vi "Log Data.vi"(6 "Edge indexies":i32[](array[numeric]), 8 "error in (no error)":errorcluster, 9 "Volatge":cdb[](array[numeric]), 10 "Frequency":dbl[](array[numeric]), 11 "Spectrum Recorder in":refnum<class "Spectrum Recorder too.lvclass">) -> (0 "error out":errorcluster, 3 "Spectrum Recorder out":refnum<class "Spectrum Recorder too.lvclass">)   [LabVIEW 2016, in "Spectrum Recorder too.lvclass"]
uses:
  Spectrum Recorder too.lvclass
  Spectrum Recorder too.lvclass/Spectrum Recorder too.ctl
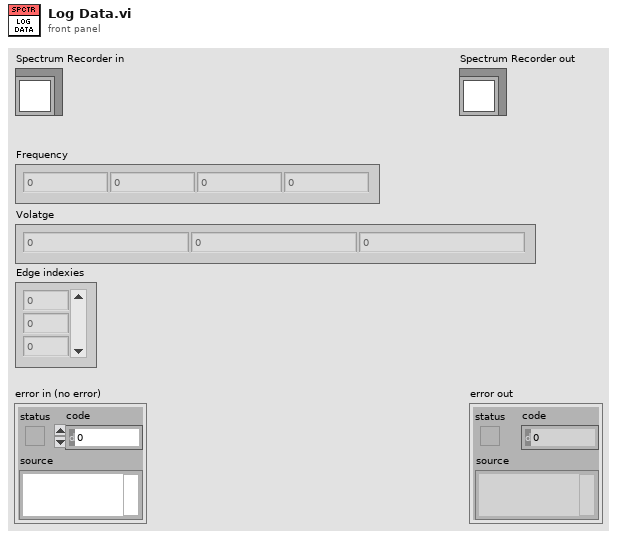
[diagram p1: front panel]
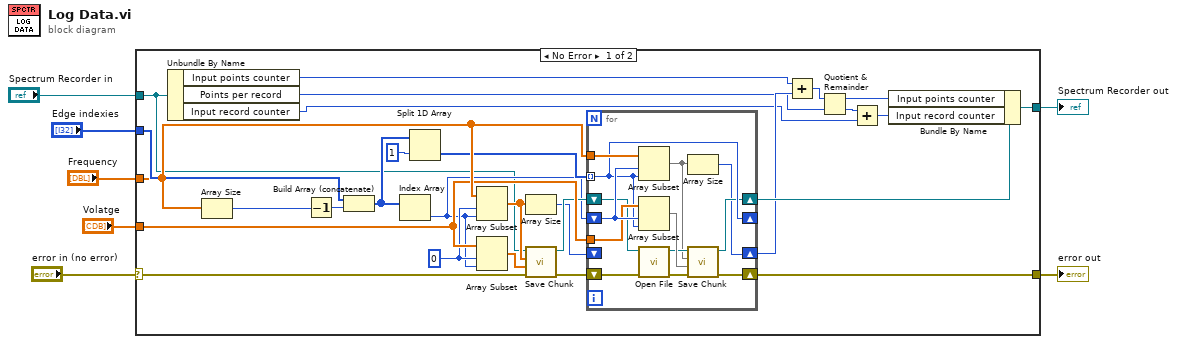
[diagram p0: block diagram]
diagram:
  n1 = case shown="No Error" "error in (no error)" {
    selector: "error in (no error)" -> [w25 w50]
    tunnel: [w31 w50] -> w6
    tunnel: [w19 w49] -> w4
    tunnel: "Spectrum Recorder in" -> [w16 w49]
    tunnel: "Edge indexies" -> [w33 _]
    tunnel: "Volatge" -> [w28 _]
    tunnel: "Frequency" -> [w29 _]
    frame No Error {
      w21 = 0
      n2 = Unbundle By Name(w16) -> ("Input points counter"=w15:i32, "Points per record"=w12:i32, "Input record counter"=w10:i32)
      n3 = Array Size(array=w29) -> (size(s)=w35:i32)
      n4 = Decrement(x=w35) -> (x-1=w34:i32)
      n5 = Build Array (concatenate)(w33, w34) -> (w27:i32[])
      n6 = Index Array(array=w27) -> (element=w20:i32)  [unwired: 1 in]
      n7 = Split 1D Array(array=w27, index=1) -> (second subarray=w23:i32[])  [unwired: 1 out]
      n8 = Array Subset(array=w29, index=w21, length=w20) -> (w17:dbl[])
      n9 = Array Subset(array=w28, index=w21, length=w20) -> (w30:cdb[])
      n10 = Array Size(array=w17) -> (size(s)=w18:i32)
      n11 = call-dynamic "Save Chunk.vi"("error in (no error)"=w25, "Voltage"=w30, "Frequency"=w17, "Spectrum Recorder in"=w16) -> ("error out"=w24:errorcluster, "Spectrum Recorder out"=w26:refnum<class "Spectrum Recorder too.lvclass">)  [unwired: 6 in]
      n12 = for {
        shift-right: [w38] -> w31
        shift-left: w24 -> [w44]
        tunnel: w29 -> [w48]
        tunnel: w28 -> [w46]
        shift-right: [w45] -> _
        shift-left: w20 -> [w47]
        tunnel: w23 -> [w45] mode=indexing
        shift-right: [w39] -> w32
        shift-left: w26 -> [w41]
        shift-right: [w37] -> w14
        shift-left: w18 -> [_]
        n13 = Array Subset(array=w48, index=w47, length=w45) -> (w36:dbl[])
        n14 = Array Subset(array=w46, index=w47, length=w45) -> (w43:cdb[])
        n15 = call-dynamic "Open File.vi"("error in (no error)"=w44, "Spectrum Recorder in"=w41) -> ("error out"=w42:errorcluster, "Spectrum Recorder out"=w40:refnum<class "Spectrum Recorder too.lvclass">)  [unwired: 8 in]
        n16 = Array Size(array=w36) -> (size(s)=w37:i32)
        n17 = call-dynamic "Save Chunk.vi"("error in (no error)"=w42, "Voltage"=w43, "Frequency"=w36, "Spectrum Recorder in"=w40) -> ("error out"=w38:errorcluster, "Spectrum Recorder out"=w39:refnum<class "Spectrum Recorder too.lvclass">)  [unwired: 6 in]
      }
      n18 = Add(x=w15, y=w14) -> (x+y=w13:i32)
      n19 = Quotient & Remainder(x=w13, y=w12) -> (x-y*floor(x/y)=w11:i32, floor(x/y)=w9:i32)
      n20 = Add(x=w9, y=w10) -> (x+y=w8:i32)
      n21 = Bundle By Name(cluster=w32, "Input points counter"=w11, "Input record counter"=w8) -> (w19:refnum<class "Spectrum Recorder too.lvclass">)
    }
    frame Error {
    }
  }
  "error out" <- w6
  "Spectrum Recorder out" <- w4
